vi "Configure Tx.vi"(0 "niUsrpRio Session":T1={"FPGA Interface"=refnum, "RIO Interface Number"=0, "Data Clock Rate"=0, "FPGA Data Clock Rate"=0, "Global Settings Register Bus"=refnum, "Radio 0 Settings Register Bus"=refnum, "Radio 1 Settings Register Bus"=refnum, "Radio Settings Bus Semaphore"=refnum, "DB Queues"=[], "Characterization Data Valid?"=FALSE, "EEPROM Header"={"Checksum"=0, "Product Code"=0, "Hardware Current Version"=0, "Hardware Oldest Compatible Version"=0, "EEPROM Map Current Version"=0, "EEPROM Map Oldest Compatible Version"=0, "User Password"="", "Pointer to Factory Header"=0, "Pointer to User Header"=0, "Recommended Interval"=0, "Number of Reserved Bytes"=9, "Number of Daughterboards"=0, "Daughterboard IDs"=[], "Daughterboard Serial Numbers"=[]}, "Device Data Header"={"Checksum"=0, "Number of Channels"=0, "Number of Gain Settings"=[], "Pointer to Characterization Data"=[], "Number of Reserved Bytes"=27, "Number of Frequencies"=[]}, "EEPROM Characterization Header"={"Checksum"=0, "Date"=timestamp(0 s since 1904-01-01), "Temperature"=0.0, "Misc. Info"="", "Pointer to Device Data Header"=0, "Number of Reserved Bytes"=28}, "Characterization Data"=[], "FPGA Current Version"=0, "FPGA Oldest Compatible Version"=0, "Fixed Logic Current Version"=0, "Fixed Logic Oldest Compatible Version"=0, "FPGA Radio Settings Bus Current Version"=0, "FPGA Radio Settings Bus Oldest Compatible Version"=0, "FPGA Board Config Current Version"=0, "FPGA Board Config Oldest Compatible Version"=0, "Daughterboard Clock Rate"=0, "daughterboard configuration session handles"=[]} {"Daughterboard Clock Rate" format="%#.3pHz"; "FPGA Data Clock Rate" format="%#.3pHz"; "Data Clock Rate" format="%#.3pHz"; "Characterization Data"."Frequencies [Hz]" format="%#_6p"; "EEPROM Characterization Header"."Pointer to Device Data Header" format="%x"; "EEPROM Characterization Header"."Checksum" format="%x"; "Device Data Header"."Pointer to Characterization Data" format="%x"; "Device Data Header"."Checksum" format="%x"; "EEPROM Header"."Pointer to User Header" format="%x"; "EEPROM Header"."Pointer to Factory Header" format="%x"; "EEPROM Header"."Product Code" format="%x"; "EEPROM Header"."Checksum" format="%x"}, 5 "tx config":T11={"channel configuration"=[], "transfer mode"=enum."Finite", "sample rate"=10000000.0, "number of samples"=8192, "start trigger"=enum."Immediate", "tone frequency"=100000.0} {"channel configuration"."channel configuration"."frequency" format="%#.3pHz"; "channel configuration"."channel configuration"."lo frequency" format="%#.3pHz"; "channel configuration"."channel configuration"."level" format="%#_gdBm"; "tone frequency" format="%#.3pHz"; "sample rate" format="%#.3pS/s"}, 7 "tx.data source":enum16{"SFP Port 0", "SFP Port 1", "Host"}(ring)=enum."Host", 11 "error in":errorcluster) -> (4 "niUsrpRio Session (out)":T1 {"Daughterboard Clock Rate" format="%#.3pHz"; "FPGA Data Clock Rate" format="%#.3pHz"; "Data Clock Rate" format="%#.3pHz"; "Characterization Data"."Frequencies [Hz]" format="%#_6p"; "EEPROM Characterization Header"."Pointer to Device Data Header" format="%x"; "EEPROM Characterization Header"."Checksum" format="%x"; "Device Data Header"."Pointer to Characterization Data" format="%x"; "Device Data Header"."Checksum" format="%x"; "EEPROM Header"."Pointer to User Header" format="%x"; "EEPROM Header"."Pointer to Factory Header" format="%x"; "EEPROM Header"."Product Code" format="%x"; "EEPROM Header"."Checksum" format="%x"}, 6 "tx.enabled channels":string[](array[string]), 8 "I":i16[](array[numeric]), 10 "Q":i16[](array[numeric]), 13 "tx.output waveform":waveform(dbl)[](graph), 14 "tx.coerced configurations":T12 {"coerced sample rates" format="%#.3pS/s"; "coerced levels" format="%#.3gdBm"; "coerced lo frequencies" format="%#.3pHz"; "coerced frequencies" format="%#.3pHz"}, 15 "error out":errorcluster)   [LabVIEW 2021]
uses:
  <instrlib>/niUsrpRio/Config/v1/Host/Public/niUsrpRio Session.ctl
  <instrlib>/_niInstr/Register Bus/v0/Host/Public/Register Bus Session.ctl
  <instrlib>/_niInstr/Register Bus/v0/Host/Private/Session Data.ctl
  <instrlib>/niUsrpRio/Config/v1/Host/Private/DB Queue Reference.ctl
  <instrlib>/niUsrpRio/Config/v1/Host/Private/Daughterboard Data.ctl
  <instrlib>/niUsrpRio/Config/v1/Host/Private/ATR state data.ctl
  <instrlib>/niUsrpRio/Config/v1/Host/Private/Antenna Configuration.ctl
  <instrlib>/niUsrpRio/Config/v1/Host/Private/CPLD Power Mode.ctl
  <instrlib>/niUsrpRio/Config/v1/Host/Public/EEPROM Header.ctl
  <instrlib>/niUsrpRio/Config/v1/Host/Public/EEPROM Device Data Header.ctl
  <instrlib>/niUsrpRio/Config/v1/Host/Public/EEPROM Characterization Header.ctl
  <instrlib>/niUsrpRio/Config/v1/Host/Public/Characterization Data.ctl
  <instrlib>/niUsrpRio/Config/v1/Host/Public/IQ Imbalance.ctl
  Start Trigger.ctl
  Configure Signal (Level).vi
  <instrlib>/_niInstr/Register Bus/v0/Host/niInstr Register Bus v0 Host.lvlib
  <instrlib>/niUsrpRio/Config/v1/Host/niUsrpRio Config v1 Host.lvlib
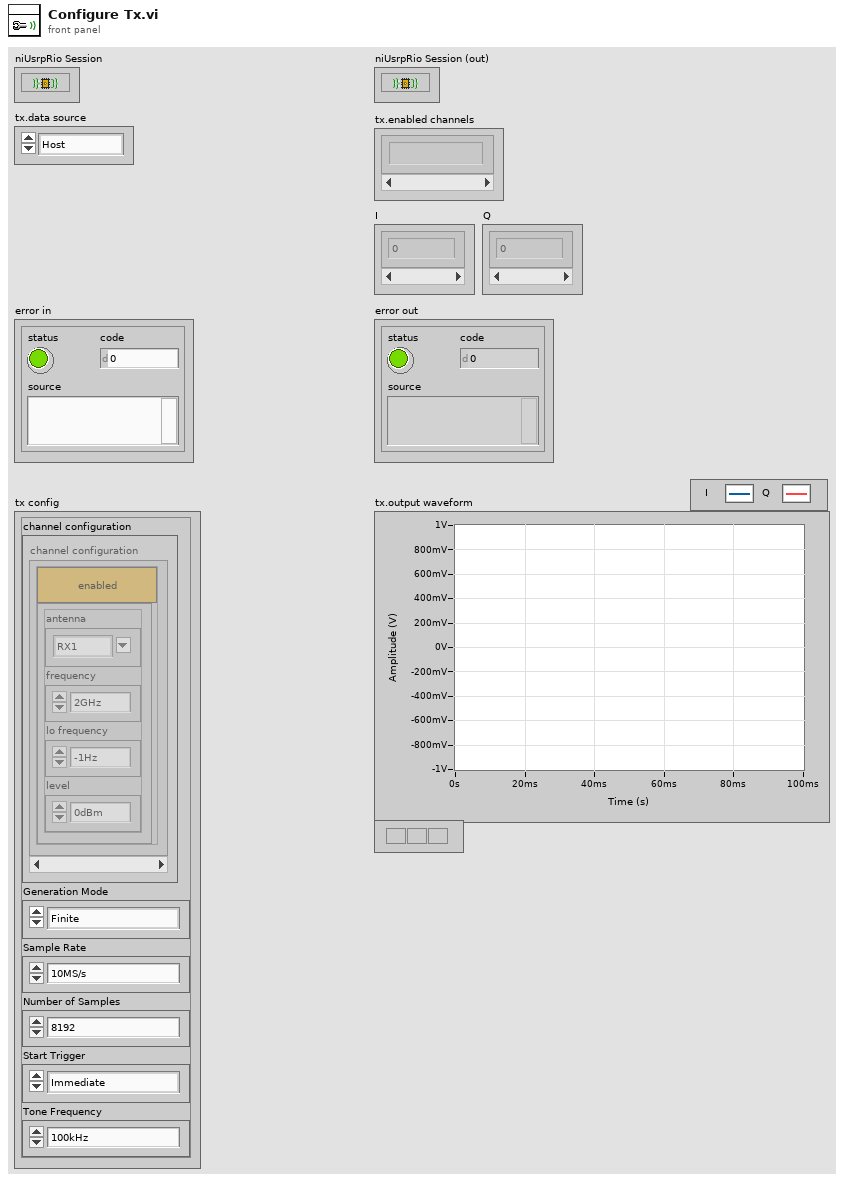
[diagram p1: front panel]
types:
  T1 = typedef "niUsrpRio Config v1 Host.lvlib/niUsrpRio Session.ctl" = cluster{"FPGA Interface":refnum<k20>, "RIO Interface Number":u32, "Data Clock Rate":u32, "FPGA Data Clock Rate":u32, "Global Settings Register Bus":T2, "Radio 0 Settings Register Bus":T2, "Radio 1 Settings Register Bus":T2, "Radio Settings Bus Semaphore":T3, "DB Queues":T4[], "Characterization Data Valid?":bool, "EEPROM Header":T5, "Device Data Header":T6, "EEPROM Characterization Header":T7, "Characterization Data":T8[], "FPGA Current Version":u32, "FPGA Oldest Compatible Version":u32, "Fixed Logic Current Version":u32, "Fixed Logic Oldest Compatible Version":u32, "FPGA Radio Settings Bus Current Version":u32, "FPGA Radio Settings Bus Oldest Compatible Version":u32, "FPGA Board Config Current Version":u32, "FPGA Board Config Oldest Compatible Version":u32, "Daughterboard Clock Rate":u32, "daughterboard configuration session handles":u64[]}
  T2 = typedef "niInstr Register Bus v0 Host.lvlib/Register Bus Session.ctl" = refnum<queue>
  T3 = typedef "Semaphore RefNum" = refnum<k1>
  T4 = typedef "niUsrpRio Config v1 Host.lvlib/DB Queue Reference.ctl" = refnum<queue>
  T5 = typedef "niUsrpRio Config v1 Host.lvlib/EEPROM Header.ctl" = cluster{"Checksum":u32, "Product Code":u16, "Hardware Current Version":u16, "Hardware Oldest Compatible Version":u16, "EEPROM Map Current Version":u16, "EEPROM Map Oldest Compatible Version":u16, "User Password":string, "Pointer to Factory Header":u32, "Pointer to User Header":u32, "Recommended Interval":u16, "Number of Reserved Bytes":i32, "Number of Daughterboards":u8, "Daughterboard IDs":u16[], "Daughterboard Serial Numbers":string[]}
  T6 = typedef "niUsrpRio Config v1 Host.lvlib/EEPROM Device Data Header.ctl" = cluster{"Checksum":u32, "Number of Channels":u8, "Number of Gain Settings":u16[], "Pointer to Characterization Data":u32[], "Number of Reserved Bytes":i32, "Number of Frequencies":u16[]}
  T7 = typedef "niUsrpRio Config v1 Host.lvlib/EEPROM Characterization Header.ctl" = cluster{"Checksum":u32, "Date":timestamp, "Temperature":sgl, "Misc. Info":string, "Pointer to Device Data Header":u32, "Number of Reserved Bytes":i32}
  T8 = typedef "niUsrpRio Config v1 Host.lvlib/Characterization Data.ctl" = cluster{"Gains[dB]":dbl[], "Frequencies [Hz]":dbl[], "IQ Imbalance Table":T9[], "Measured Gains[dB]":dbl[][]}
  T9 = typedef "niUsrpRio Config v1 Host.lvlib/IQ Imbalance.ctl" = cluster{"Gain Imbalance [linear]":dbl, "Phase Imbalance [radians]":dbl, "Offset":cdb}
  T10 = typedef "Start Trigger.ctl" = enum8{"Software", "Digital Edge", "Rx Start Trigger", "Tx Start Trigger", "Immediate", "Future Time Event"}
  T11 = cluster{"channel configuration":cluster{"channel enable":bool, "channel configuration":cluster{"antenna":string, "frequency":dbl, "lo frequency":dbl, "level":dbl}}[], "transfer mode":enum16{"Finite", "Continuous"}, "sample rate":dbl, "number of samples":u32, "start trigger":T10, "tone frequency":dbl}
  T12 = cluster{"coerced frequencies":dbl[], "coerced lo frequencies":dbl[], "coerced levels":dbl[], "coerced sample rates":dbl[]}
  T13 = cluster{"channel enable":bool, "channel configuration":cluster{"antenna":string, "frequency":dbl, "lo frequency":dbl, "level":dbl}}[]
  T14 = cluster{"antenna":string, "frequency":dbl, "lo frequency":dbl, "level":dbl}[]
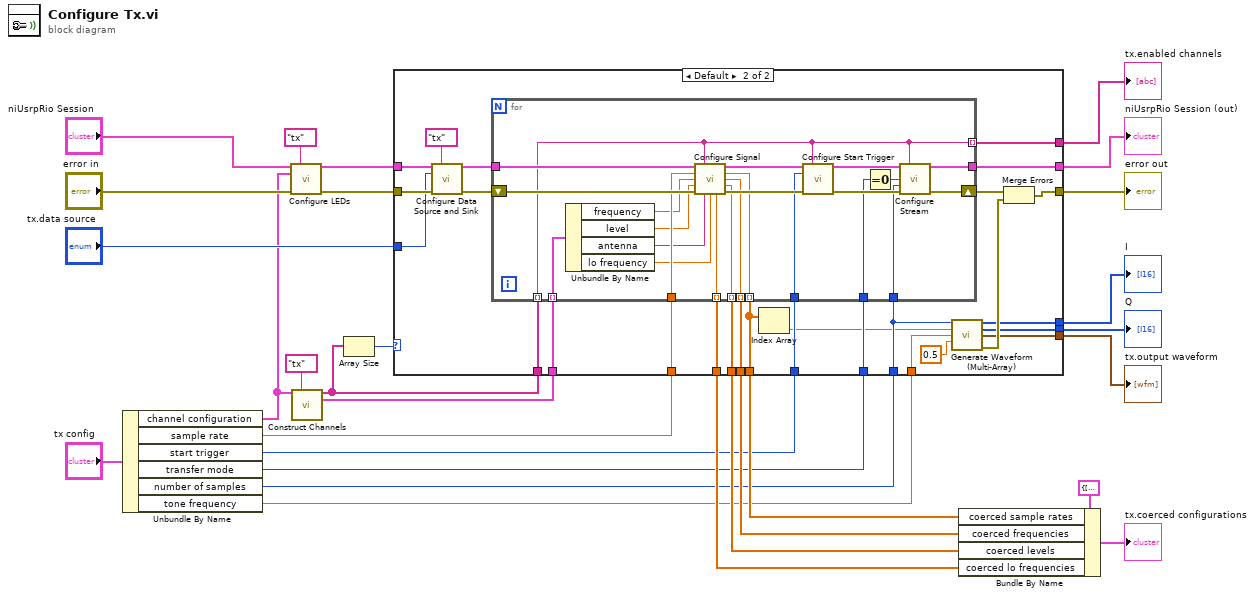
[diagram p0: block diagram]
diagram:
  n1 = Unbundle By Name("tx config") -> ("channel configuration"=w1:T13, "sample rate"=w11:dbl, "start trigger"=w10:T10, "transfer mode"=w9:enum16{"Finite", "Continuous"}, "number of samples"=w8:u32, "tone frequency"=w7:dbl)
  n2 = call "Configure LEDs.vi"("niUsrpRio Session"="niUsrpRio Session", "scope"="tx", "channel configurations"=w1, "error in"="error in") -> ("niUsrpRio Session (out)"=w3:T1, "error out"=w6:errorcluster)  [unwired: 10 in]
  n3 = call "Construct Channels.vi"("channel configurations"=w1, "scope"="tx") -> ("enabled channels"=w17:string[], "enabled channel configurations"=w24:T14)  [unwired: 12 in]
  n4 = Array Size(array=w17) -> (size(s)=w18:i32)
  n5 = case shown="Default" w18 {
    tunnel: [_ w39] -> w29
    tunnel: [_ w58] -> w28
    tunnel: [_ w57] -> w27
    tunnel: [_ w56] -> w26
    tunnel: w10 -> [_ w55]
    tunnel: w17 -> [_ w54]
    tunnel: w24 -> [_ w53]
    tunnel: [_ w52] -> w23
    tunnel: w11 -> [_ w47]
    tunnel: w9 -> [_ w51]
    tunnel: w8 -> [_ w46]
    tunnel: [w31 w50] -> w19
    tunnel: w6 -> [w30 w35]
    tunnel: w3 -> [w31 w37]
    tunnel: [w30 w44] -> w25
    tunnel: w7 -> [_ w48]
    tunnel: [_ w42] -> w16
    tunnel: [_ w41] -> w15
    tunnel: [_ w40] -> w14
    tunnel: "tx.data source" -> [_ w33]
    frame 0 {
    }
    frame Default {
      n6 = call "Configure Data Source and Sink.vi"("niUsrpRio Session"=w37, "scope"="tx", "data stream config"=w33, "error in"=w35) -> ("niUsrpRio Session (out)"=w36:T1, "error out"=w34:errorcluster)  [unwired: 10 in]
      n7 = for "channel configuration" {
        tunnel: [w75] -> w56 mode=indexing
        tunnel: w55 -> [w77]
        tunnel: w46 -> [w61]
        tunnel: w51 -> [w76]
        shift-right: [w60] -> w49
        shift-left: w34 -> [w81]
        tunnel: w47 -> [w80]
        tunnel: [w74] -> w57 mode=indexing
        tunnel: [w73] -> w58 mode=indexing
        tunnel: [w72] -> w39 mode=indexing
        tunnel: w53 -> [w71] mode=indexing
        tunnel: w54 -> [w68] mode=indexing
        tunnel: [w68] -> w52 mode=indexing
        tunnel: [w70] -> w50
        tunnel: w36 -> [w69]
        n8 = Unbundle By Name(w71) -> ("frequency"=w65:dbl, "level"=w62:dbl, "antenna"=w64:string, "lo frequency"=w63:dbl)
        n9 = call-poly "Configure Signal.vi"("niUsrpRio Session"=w69, "scope"=w68, "sample rate [S/s]"=w80, "frequency [Hz]"=w65, "level [dBm]"=w62, "error in"=w81, "Active Antenna"=w64, "LO frequency [Hz]"=w63) -> ("niUsrpRio Session (out)"=w67:T1, "coerced sample rate [S/s]"=w72:dbl, "coerced frequency [Hz]"=w73:dbl, "coerced level [dBm]"=w74:dbl, "coerced LO frequency [Hz]"=w75:dbl, "error out"=w79:errorcluster)  [unwired: 1 in, 1 out]
        n10 = call "Configure Start Trigger.vi"("niUsrpRio Session"=w67, "scope"=w68, "start trigger"=w77, "error in"=w79) -> ("niUsrpRio Session (out)"=w66:T1, "error out"=w78:errorcluster)  [unwired: 10 in]
        n11 = Equal To 0?(x=w76) -> (x = 0?=w59:bool)
        n12 = call "Configure Stream.vi"("niUsrpRio Session"=w66, "scope"=w68, "number of samples is finite"=w59, "number of samples"=w61, "error in"=w78) -> ("niUsrpRio Session (out)"=w70:T1, "error out"=w60:errorcluster)  [unwired: 9 in]
      }
      n13 = Index Array(array=w39) -> (element=w38:dbl)  [unwired: 1 in]
      n14 = call "Generate Waveform (Multi-Array).vi"("number of samples"=w46, "sample rate"=w38, "tone frequency"=w48, "amplitude"=0.5) -> ("I"=w42:i16[], "Q"=w41:i16[], "Waveform"=w40:waveform(dbl)[], "error out"=w43:errorcluster)  [unwired: 8 in]
      n15 = Merge Errors(w49, w43) -> (w44:errorcluster)
    }
  }
  "niUsrpRio Session (out)" <- w19
  "error out" <- w25
  "tx.enabled channels" <- w23
  "tx.output waveform" <- w14
  "I" <- w16
  "Q" <- w15
  n16 = Bundle By Name(cluster=T12 {"coerced frequencies"=[], "coerced lo frequencies"=[], "coerced levels"=[], "coerced sample rates"=[]} ("coerced configurations"), "coerced sample rates"=w29, "coerced frequencies"=w28, "coerced levels"=w27, "coerced lo frequencies"=w26) -> (→"tx.coerced configurations":T12)
